vi "MRU_Destroy.vi"(8 "error in (no error)":errorcluster, 11 "reference in":refnum<class "MRU.lvclass">) -> (0 "error out":errorcluster, 3 "reference out":refnum<class "MRU.lvclass">)   [LabVIEW 2014, in "MRU.lvclass"]
doc: "Cleans up the MRU Object. This should be called when you are finished with the MRU Object."
uses:
  MRU.lvclass
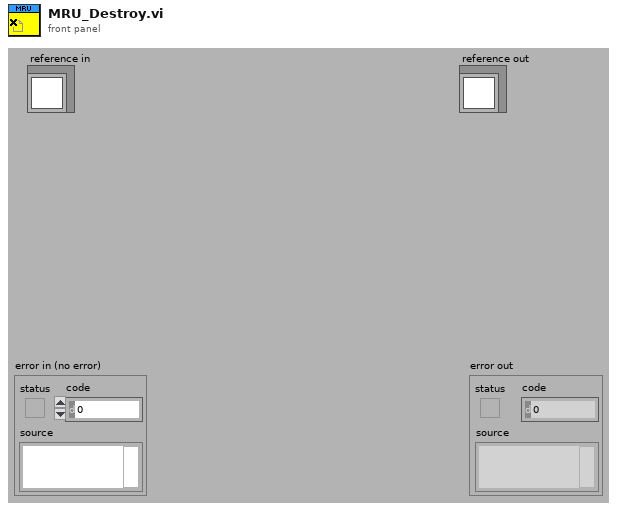
[diagram p1: front panel]
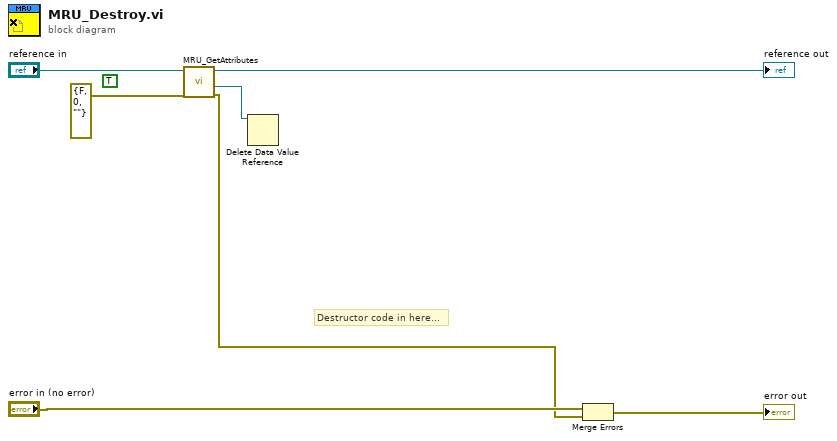
[diagram p0: block diagram]
diagram:
  (unwired) TRUE ("Simple Info")
  # "Destructor code in here..."
  n1 = call "MRU_GetAttributes.vi"("error in (no error)"=errorcluster {"status"=FALSE, "code"=0, "source"=""}, "reference in"="reference in") -> ("error out"=w5:errorcluster, "DataRef"=w1:refnum<data-value>, "reference out"=→"reference out":refnum<class "MRU.lvclass">)  [unwired: 1 in, 6 out]
  n2 = Delete Data Value Reference(data value reference=w1) -> ()  [unwired: 1 in, 2 out]
  n3 = Merge Errors("error in (no error)", w5) -> (→"error out":errorcluster)
